vi "Read Clock Discipline.vi"(8 "error in (no error)":errorcluster, 11 "RT Data Cluster in":T1={"Timekeeper hdl"="", "clkDisc session"=variant, "Compiled Data"={"SyncMod?"=FALSE, "SyncMod"="", "ConnectionSettings"={"Mode"=enum."Generate sample clock", "pxitrig"=FALSE, "pfi0"=FALSE, "pfi1"=FALSE, "pfi2"=FALSE, "External Pin"=enum."PFI0", "Routes"=[]}, "TimeKeeper"="", "ScanOffset(%)"=0.0, "StartDelay(s)"=0, "Time Ref Settings"={"Time Reference"=enum."GPS", "Priority 1"=0, "Priority 2"=0, "IRIG type"=enum."IRIGB AM", "Terminal"="", "PPSSetTime"=FALSE, "Start Time"=timestamp(0 s since 1904-01-01)}, "FIFO Locations"={"SysTime"=[], "TimeRef"=[], "Status"=[]}}, "OutputsData"=[], "OutputsFIFO"=refnum, "Scan Period"=0, "Timekeeper type"=enum."6683", "SyncMod type"=enum."6683", "SyncMod hdl"=""} {"Compiled Data"."Time Ref Settings"."Priority 2" min=0 max=255; "Compiled Data"."Time Ref Settings"."Priority 1" min=0 max=255}) -> (0 "error out":errorcluster, 3 "RT Data Cluster out":T1={"Timekeeper hdl"="", "clkDisc session"=variant, "Compiled Data"={"SyncMod?"=FALSE, "SyncMod"="", "ConnectionSettings"={"Mode"=enum."Generate sample clock", "pxitrig"=FALSE, "pfi0"=FALSE, "pfi1"=FALSE, "pfi2"=FALSE, "External Pin"=enum."PFI0", "Routes"=[]}, "TimeKeeper"="", "ScanOffset(%)"=0.0, "StartDelay(s)"=0, "Time Ref Settings"={"Time Reference"=enum."GPS", "Priority 1"=0, "Priority 2"=0, "IRIG type"=enum."IRIGB AM", "Terminal"="", "PPSSetTime"=FALSE, "Start Time"=timestamp(0 s since 1904-01-01)}, "FIFO Locations"={"SysTime"=[], "TimeRef"=[], "Status"=[]}}, "OutputsData"=[], "OutputsFIFO"=refnum, "Scan Period"=0, "Timekeeper type"=enum."6683", "SyncMod type"=enum."6683", "SyncMod hdl"=""} {"Compiled Data"."Time Ref Settings"."Priority 2" min=0 max=255; "Compiled Data"."Time Ref Settings"."Priority 1" min=0 max=255}, 5 "Sync":bool)   [LabVIEW 2018, in "Chassis TimeSync Engine.lvlib"]
uses:
  Chassis TimeSync Engine.lvlib
  RT Data Cluster.ctl
  mdevClkDisc.llb/_clkDisc_session.ctl
  Shared/Compiled Data.ctl
  Shared/Connection Settings.ctl
  Shared/Mode.ctl
  Shared/External Pin.ctl
  Shared/Routes.ctl
  Shared/Route.ctl
  Shared/Time Ref Settings.ctl
  Shared/Time Reference.ctl
  Shared/IRIG Type.ctl
  timekeeper type.ctl
  Shared/Chassis TimeSync Shared.lvlib
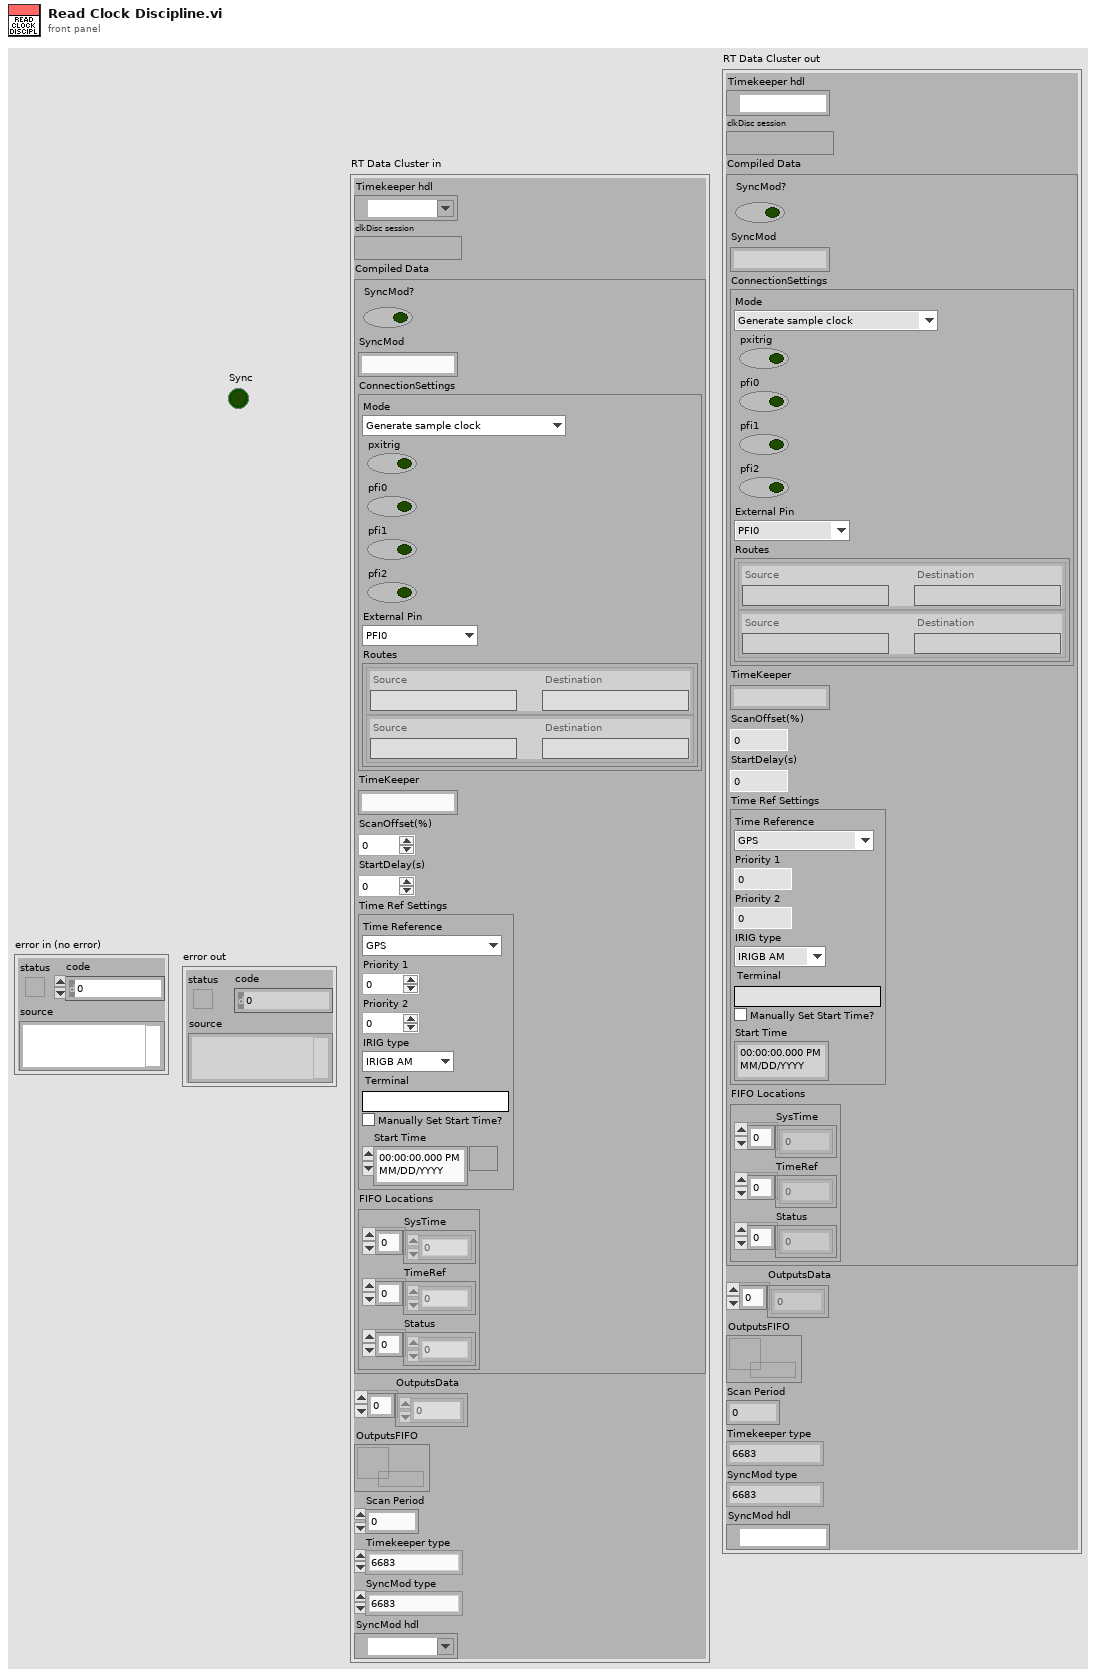
[diagram p1: front panel]
types:
  T1 = typedef "Chassis TimeSync Engine.lvlib/RT Data Cluster.ctl" = cluster{"Timekeeper hdl":refnum<k15>, "clkDisc session":T2, "Compiled Data":T3, "OutputsData":dbl[], "OutputsFIFO":refnum<k33>, "Scan Period":u32, "Timekeeper type":T12, "SyncMod type":T12, "SyncMod hdl":refnum<k15>}
  T2 = typedef "_clkDisc_session.ctl" = variant
  T3 = typedef "Chassis TimeSync Shared.lvlib/Compiled Data.ctl" = cluster{"SyncMod?":bool, "SyncMod":string, "ConnectionSettings":T4, "TimeKeeper":string, "ScanOffset(%)":dbl, "StartDelay(s)":u16, "Time Ref Settings":T9, "FIFO Locations":cluster{"SysTime":i32[], "TimeRef":i32[], "Status":i32[]}}
  T4 = typedef "Chassis TimeSync Shared.lvlib/Connection Settings.ctl" = cluster{"Mode":T5, "pxitrig":bool, "pfi0":bool, "pfi1":bool, "pfi2":bool, "External Pin":T6, "Routes":T7}
  T5 = typedef "Chassis TimeSync Shared.lvlib/Mode.ctl" = enum16{"Generate sample clock", "Route sample clock out of chassis", "Route sample clock into chassis", "Custom routes"}
  T6 = typedef "Chassis TimeSync Shared.lvlib/External Pin.ctl" = enum16{"PFI0", "PFI1", "PFI2"}
  T7 = typedef "Chassis TimeSync Shared.lvlib/Routes.ctl" = T8[]
  T8 = typedef "Chassis TimeSync Shared.lvlib/Route.ctl" = cluster{"Source":string, "Destination":string}
  T9 = typedef "Chassis TimeSync Shared.lvlib/Time Ref Settings.ctl" = cluster{"Time Reference":T10, "Priority 1":i32, "Priority 2":i32, "IRIG type":T11, "Terminal":string, "PPSSetTime":bool, "Start Time":timestamp}
  T10 = typedef "Chassis TimeSync Shared.lvlib/Time Reference.ctl" = enum16{"GPS", "IRIG", "PPS", "1588 Ordinary Clock", "PXI Chassis Clock", "Free Running (Internal)"}
  T11 = typedef "Chassis TimeSync Shared.lvlib/IRIG Type.ctl" = enum16{"IRIGB DC", "IRIGB AM"}
  T12 = typedef "Chassis TimeSync Engine.lvlib/timekeeper type.ctl" = enum16{"6683", "6683H", "6682", "6682H", "non-timekeeper", "timekeeper"}
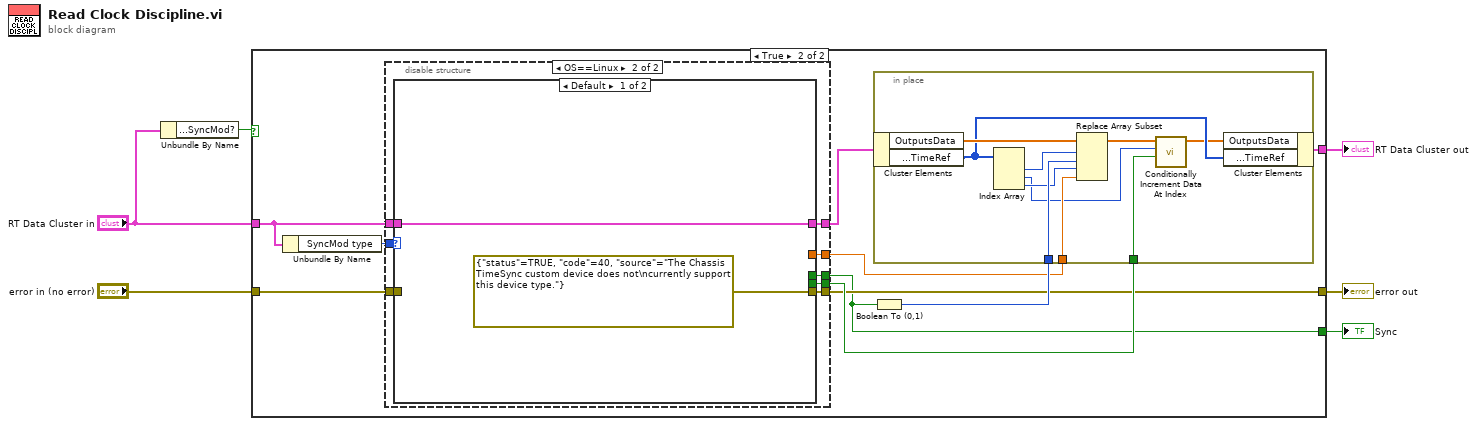
[diagram p0: block diagram]
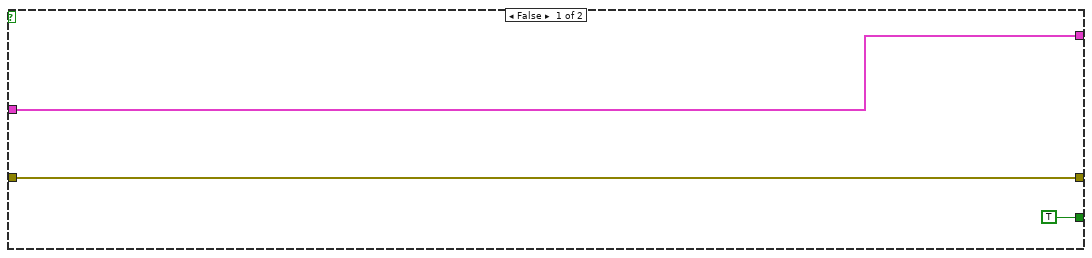
[diagram p2: hidden frame]
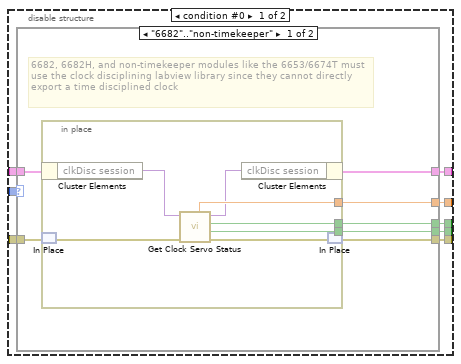
[diagram p3: hidden frame]
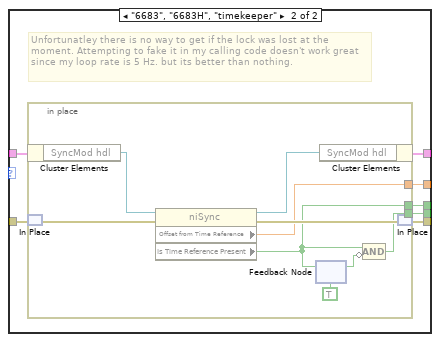
[diagram p4: hidden frame]
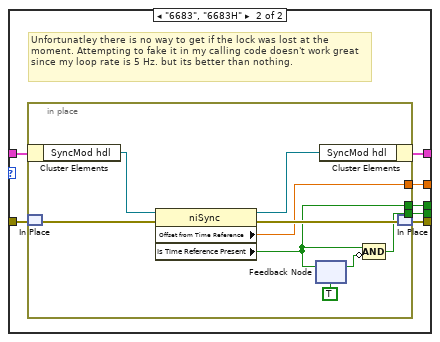
[diagram p5: hidden frame]
diagram:
  n1 = Unbundle By Name("RT Data Cluster in") -> ("Compiled Data.SyncMod?"=w2:bool)
  n2 = case shown="True" w2 {
    tunnel: [w8 w19] -> w6
    tunnel: "error in (no error)" -> [w9 w15]
    tunnel: [w9 w13] -> w4
    tunnel: "RT Data Cluster in" -> [w8 w11]
    tunnel: [TRUE ("Servo Locked") w12] -> w1
    frame False {
    }
    frame True {
      n3 = Unbundle By Name(w11) -> ("SyncMod type"=w10:T12)
      n4 = disable-structure shown="OS==Linux" {
        disable-tunnel: [w27 w65] -> w17
        disable-tunnel: [w26 w64] -> w16
        disable-tunnel: w15 -> [w25 w63]
        disable-tunnel: [w24 w62] -> w14
        disable-tunnel: [w23 w61] -> w13
        disable-tunnel: [w22 w60] -> w12
        disable-tunnel: w11 -> [w21 w59]
        disable-tunnel: w10 -> [w20 w58]
        frame condition #0 {
          n5 = case shown="\"6682\"..\"non-timekeeper\"" w20 {
            tunnel: [w34 w48] -> w27
            tunnel: [w33 w47] -> w26
            tunnel: w25 -> [w32 w46]
            tunnel: [w31 w45] -> w24
            tunnel: [w30 w44] -> w23
            tunnel: [w29 w43] -> w22
            tunnel: w21 -> [w28 w42]
            frame "6682".."non-timekeeper" {
              # "6682, 6682H, and non-timekeeper modules like the 6653/6674T must use the clock disciplining labview library since they cannot directly export a time disciplined clock"
              n6 = in-place {
                in-place-border: [w41] -> w29
                in-place-border: [w40] -> w34
                in-place-border: [w39] -> w33
                n7 = in-place-cluster #1(w28) -> ("clkDisc session"=w36:T2)
                n8 = in-place-match #2(w32) -> (w38:errorcluster)
                n9 = call "Get Clock Servo Status.vi"("clkDisc session (in)"=w36, "error out"=w38) -> ("Calculated Time Reference Offset"=w39:dbl, "clkDisc session (out)"=w35:T2, "Servo Locked"=w41:bool, "Servo Lock Lost"=w40:bool, "error (out)"=w37:errorcluster)  [unwired: 2 in]
                n10 = in-place-cluster #1("clkDisc session"=w35) -> (w31:T1)
                n11 = in-place-match #2(w37) -> (w30:errorcluster)
              }
            }
            frame "6683", "6683H", "timekeeper" {
              # "Unfortunatley there is no way to get if the lock was lost at the moment. Attempting to fake it in my calling code doesn't work great since my loop rate is 5 Hz. but its better than nothing."
              n12 = in-place {
                in-place-border: [w50] -> w43
                in-place-border: [w49] -> w48
                in-place-border: [w53] -> w47
                n13 = in-place-cluster #3(w42) -> ("SyncMod hdl"=w56:refnum<k15>)
                n14 = in-place-match #4(w46) -> (w57:errorcluster)
                n15 = property class="niSync"(reference=w56, error in=w57) -> (reference out=w55:refnum<k15>, error out=w54:errorcluster, "Offset from Time Reference"=w53:dbl, "Is Time Reference Present"=w50:bool)
                n16 = feedback-in #5(w50) -> ()
                n17 = feedback #5(TRUE) -> (w51:bool)
                n18 = in-place-cluster #3("SyncMod hdl"=w55) -> (w45:T1)
                n19 = Compound Arithmetic op=AND(w50, invert w51) -> (w49:bool)
                n20 = in-place-match #4(w54) -> (w44:errorcluster)
              }
            }
          }
        }
        frame condition #1 (active) {
          n21 = case shown="Default" w58 {
            tunnel: [_ w74] -> w65
            tunnel: [_ w73] -> w64
            tunnel: w63 -> [_ w72]
            tunnel: [w66 w71] -> w62
            tunnel: [errorcluster {"status"=TRUE, "code"=40, "source"="The Chassis TimeSync custom device does not\ncurrently support this device type."} ("error out") w70] -> w61
            tunnel: [_ w69] -> w60
            tunnel: w59 -> [w66 w68]
            frame Default {
            }
            frame "6683", "6683H" {
              # "Unfortunatley there is no way to get if the lock was lost at the moment. Attempting to fake it in my calling code doesn't work great since my loop rate is 5 Hz. but its better than nothing."
              n22 = in-place {
                in-place-border: [w76] -> w69
                in-place-border: [w75] -> w74
                in-place-border: [w79] -> w73
                n23 = in-place-cluster #6(w68) -> ("SyncMod hdl"=w82:refnum<k15>)
                n24 = in-place-match #7(w72) -> (w83:errorcluster)
                n25 = property class="niSync"(reference=w82, error in=w83) -> (reference out=w81:refnum<k15>, error out=w80:errorcluster, "Offset from Time Reference"=w79:dbl, "Is Time Reference Present"=w76:bool)
                n26 = feedback-in #8(w76) -> ()
                n27 = feedback #8(TRUE) -> (w77:bool)
                n28 = in-place-cluster #6("SyncMod hdl"=w81) -> (w71:T1)
                n29 = Compound Arithmetic op=AND(w76, invert w77) -> (w75:bool)
                n30 = in-place-match #7(w80) -> (w70:errorcluster)
              }
            }
          }
        }
      }
      n31 = Boolean To (0,1)(Boolean=w12) -> (0, 1=w18:i16)
      n32 = in-place {
        in-place-border: w16 -> [w89]
        in-place-border: w18 -> [w90]
        in-place-border: w17 -> [w84]
        n33 = in-place-cluster #9(w14) -> ("OutputsData"=w93:dbl[], "Compiled Data.FIFO Locations.TimeRef"=w91:i32[])
        n34 = Index Array(array=w91) -> (element #1=w92:i32, element #2=w85:i32, element #3=w88:i32)  [unwired: 3 in]
        n35 = Replace Array Subset(array=w93, new element #1=w90, index #1=w92, new element #2=w89, index #2=w88) -> (w87:dbl[])
        n36 = call "Conditionally Increment Data At Index.vi"("Increment"=w84, "Data index"=w85, "Data in"=w87) -> ("Data out"=w86:dbl[])  [unwired: 8 in]
        n37 = in-place-cluster #9("OutputsData"=w86, "Compiled Data.FIFO Locations.TimeRef"=w91) -> (w19:T1)
      }
    }
  }
  "error out" <- w4
  "RT Data Cluster out" <- w6
  "Sync" <- w1
